vi "4kWaveformFilter.vi"(9 "Low cutoff":dbl=4000.0, 10 "High cutoff":dbl=150000.0, 11 "data":waveform(dbl)) -> (3 "Waveform":waveform(dbl))   [LabVIEW 2017]
uses:
  <vilib>/Analysis/3filter.llb/Elliptic Filter (DBL).vi
  <vilib>/Analysis/NI_AALBase.lvlib
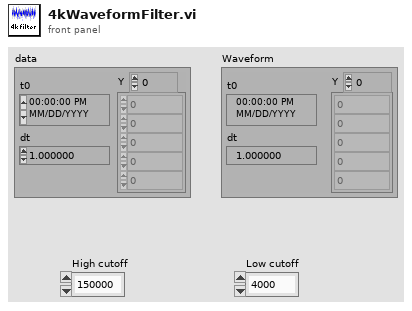
[diagram p1: front panel]
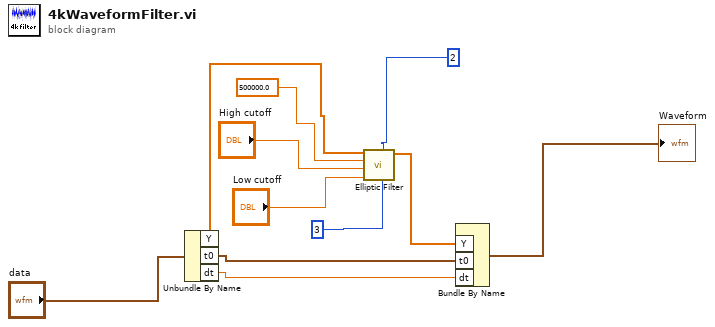
[diagram p0: block diagram]
diagram:
  n1 = Unbundle By Name("data") -> ("Y"=w1:dbl[], "t0"=w9:timestamp, "dt"=w10:dbl)
  n2 = call-poly <vilib>:"Elliptic Filter.vi"("order"=3, "filter type"=2, "low cutoff freq: fl"="Low cutoff", "high cutoff freq: fh"="High cutoff", "sampling freq: fs"=500000.0, "X"=w1) -> ("Filtered X"=w6:dbl[])  [unwired: 4 in, 1 out]
  n3 = Bundle By Name("Y"=w6, "t0"=w9, "dt"=w10) -> (→"Waveform":waveform(dbl))  [unwired: 1 in]
